vi "LEDSA Loop --0 IO--.vi"(2 "Error In":errorcluster, 3 "FPGA VI Reference In":refnum<k20>) -> (0 "Error Out":errorcluster, 1 "FPGA VI Reference Out":refnum<k20>)   [LabVIEW 2015]
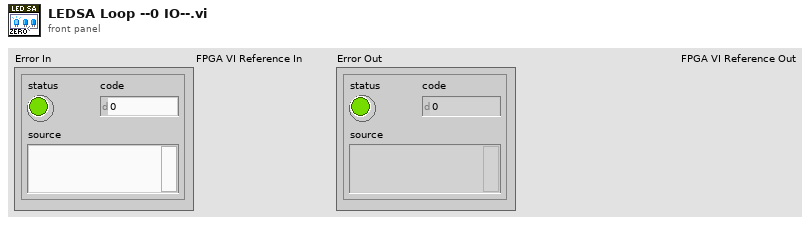
[diagram p1: front panel]
types:
  T1 = cluster{"LED 3":enum16{"Brightness", "Bool"}, "BOOL":bool, "Brightness":u32}
  T2 = cluster{"LED 1":enum16{"Brightness", "Bool"}, "BOOL":bool, "Brightness":u32}
  T3 = cluster{"LED 2":enum16{"Brightness", "Bool"}, "BOOL":bool, "Brightness":u32}
  T4 = cluster{"LED 0":enum16{"Brightness", "Bool"}, "BOOL":bool, "Brightness":u32}
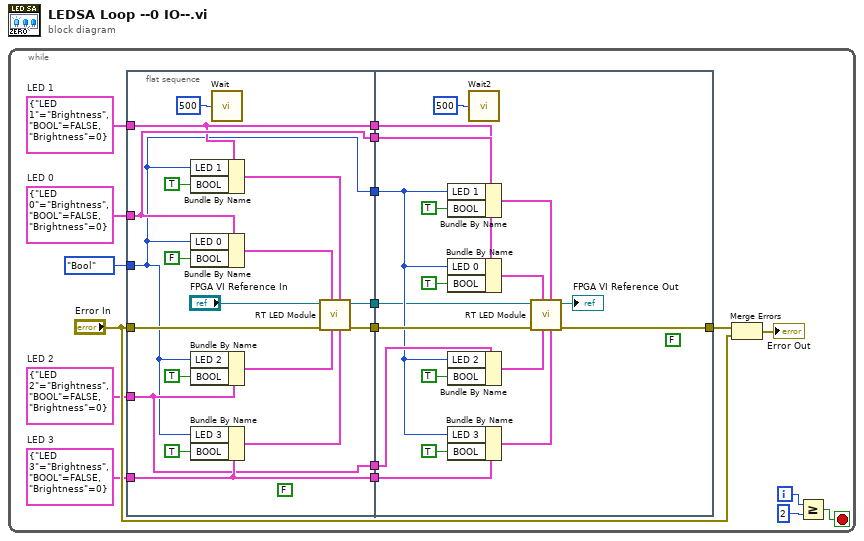
[diagram p0: block diagram]
diagram:
  n1 = while {
    i -> [w14]
    stop <- w12 stop-if-true
    w6 = T1 {"LED 3"=enum."Brightness", "BOOL"=FALSE, "Brightness"=0}  # LED 3
    w4 = T2 {"LED 1"=enum."Brightness", "BOOL"=FALSE, "Brightness"=0}  # LED 1
    w5 = T3 {"LED 2"=enum."Brightness", "BOOL"=FALSE, "Brightness"=0}  # LED 2
    w11 = T4 {"LED 0"=enum."Brightness", "BOOL"=FALSE, "Brightness"=0}  # LED 0
    n2 = flat-sequence {
      tunnel: "Error In" -> [w35]
      tunnel: [w34] -> w18
      tunnel: w11 -> [w33]
      tunnel: [w33] -> w10
      tunnel: [w32] -> w9
      tunnel: [w31] -> w8
      tunnel: [w30] -> w7
      tunnel: w6 -> [w32]
      tunnel: w5 -> [w31]
      tunnel: w4 -> [w30]
      tunnel: enum16{"Brightness", "Bool"}."Bool" ("LED") -> [w29]
      tunnel: [w29] -> w2
      tunnel: [w24] -> w1
      tunnel: w18 -> [w53]
      tunnel: [w52] -> w17
      tunnel: w10 -> [w51]
      tunnel: w9 -> [w50]
      tunnel: w8 -> [w49]
      tunnel: w7 -> [w48]
      tunnel: w2 -> [w47]
      tunnel: w1 -> [w42]
      frame #0 {
        (unwired) FALSE ("Stop Button")
        n3 = Bundle By Name(cluster=w30, "LED 1"=w29, "BOOL"=TRUE ("LED 1")) -> (w22:T2)
        n4 = Bundle By Name(cluster=w33, "LED 0"=w29, "BOOL"=FALSE ("LED 0")) -> (w20:T4)
        n5 = Bundle By Name(cluster=w31, "LED 2"=w29, "BOOL"=TRUE ("LED 2")) -> (w23:T3)
        n6 = Bundle By Name(cluster=w32, "LED 3"=w29, "BOOL"=TRUE ("LED 3")) -> (w21:T1)
        n7 = call "Wait"("Count(mSec)"=u32 500) -> ()  [unwired: 1 out]
        n8 = call "RT LED Module.vi"("LED 3"=w21, "LED 1"=w22, "LED 2"=w23, "LED 0"=w20, "error in"=w35, "FPGA VI Reference In"="FPGA VI Reference In") -> ("error out"=w34:errorcluster, "FPGA VI Reference Out"=w24:refnum<k20>)  [unwired: 4 in]
      }
      frame #1 {
        (unwired) FALSE ("Stop Button")
        n9 = Bundle By Name(cluster=w48, "LED 1"=w47, "BOOL"=TRUE ("LED 2")) -> (w39:T2)
        n10 = Bundle By Name(cluster=w51, "LED 0"=w47, "BOOL"=TRUE ("LED 3")) -> (w41:T4)
        n11 = Bundle By Name(cluster=w49, "LED 2"=w47, "BOOL"=TRUE ("LED 0")) -> (w38:T3)
        n12 = Bundle By Name(cluster=w50, "LED 3"=w47, "BOOL"=TRUE ("LED 1")) -> (w40:T1)
        n13 = call "Wait2"("Count(mSec)"=u32 500) -> ()  [unwired: 1 out]
        n14 = call "RT LED Module.vi"("LED 3"=w40, "LED 1"=w39, "LED 2"=w38, "LED 0"=w41, "error in"=w53, "FPGA VI Reference In"=w42) -> ("error out"=w52:errorcluster, "FPGA VI Reference Out"=→"FPGA VI Reference Out":refnum<k20>)  [unwired: 4 in]
      }
    }
    n15 = Merge Errors(w17, "Error In") -> (→"Error Out":errorcluster)
    n16 = Greater Or Equal?(x=w14, y=2) -> (x >= y?=w12:bool)
  }
